vi "Reentrant Method.vi"(8 "error in (no error)":errorcluster, 10 "Numeric":dbl, 11 "Test Interface Mock in":refnum<class "Test Interface Responsive Mock.lvclass">) -> (0 "error out":errorcluster, 3 "Test Interface Mock out":refnum<class "Test Interface Responsive Mock.lvclass">)   [LabVIEW 2020, in "Test Interface Responsive Mock.lvclass"]
uses:
  Test Interface Responsive Mock.lvclass
  C:/git/astemes-lmock/source/Framework/Responsive Mock/Responsive Mock.lvclass
  source/Framework/Responsive Mock/Responsive Mock.lvclass/Responsive Mock.ctl
  <vilib>/Utility/error.llb/Clear Errors.vi
  source/Framework/Parametric VI Call/Parametric VI Call.lvclass
  C:/git/astemes-lmock/source/Core/VI Call/VI Call.lvclass
  source/Framework/Parametric VI Call/Create.vi
  source/Core/Expectation/Expectation.lvclass
  Test Interface Responsive Mock.lvclass/Test Interface Responsive Mock.ctl
  source/Framework/Responsive Mock/Responsive Mock.lvclass
panel:
  # "IMPORTANT!"
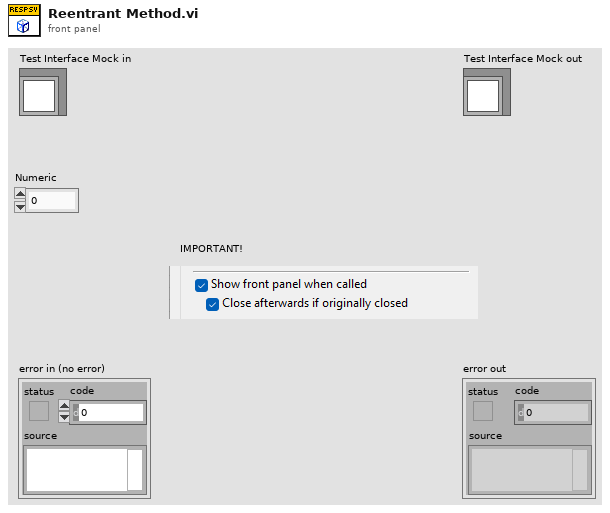
[diagram p1: front panel]
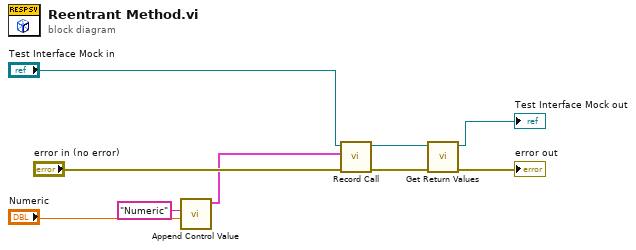
[diagram p0: block diagram]
diagram:
  n1 = call "Append Control Value.vi"("Variant Data"="Numeric", "Name"="Numeric") -> ("Control Values"=w4:cluster{"Name":string, "Variant Data":variant}[])  [unwired: 9 in]
  n2 = call "Record Call.vi"("error in (no error)"="error in (no error)", "Control Values"=w4, "Mock In"="Test Interface Mock in") -> ("error out"=w8:errorcluster, "Mock Out"=w2:refnum<class "Test Interface Responsive Mock.lvclass">)  [unwired: 7 in]
  n3 = call "Get Return Values.vi"("error in (no error)"=w8, "Mock In"=w2) -> ("error out"=→"error out":errorcluster, "Mock Out"=→"Test Interface Mock out":refnum<class "Test Interface Responsive Mock.lvclass">)  [unwired: 7 in, 1 out]
